vi "TCP-Get Status.vi"(0 "IP Address":string, 5 "Port":i32, 11 "error in (no error)":errorcluster) -> (4 "Recording":bool, 15 "error out":errorcluster)   [LabVIEW 2020]
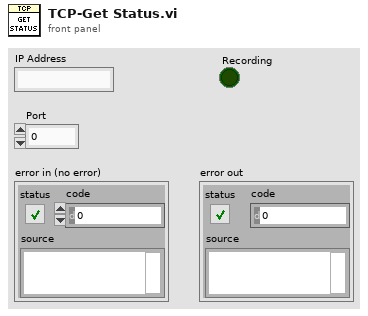
[diagram p1: front panel]
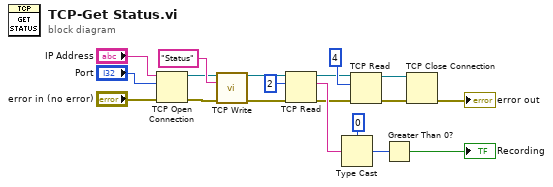
[diagram p0: block diagram]
diagram:
  n1 = TCP Open Connection(address="IP Address", remote port or service name="Port", error in (no error)="error in (no error)") -> (connection ID=w4:refnum<k5>, error out=w3:errorcluster)  [unwired: 2 in]
  n2 = call "TCP Write.vi"("connection ID"=w4, "data string"="Status", "error in (no error)"=w3) -> ("connection ID out"=w7:refnum<k5>, "error out"=w6:errorcluster)  [unwired: 10 in, 1 out]
  n3 = TCP Read(connection ID=w7, bytes to read=2, error in (no error)=w6) -> (connection ID out=w11:refnum<k5>, data out=w12:string, error out=w10:errorcluster)  [unwired: 2 in]
  n4 = Type Cast(type=i16 0, x=w12) -> (*(type *) &x=w17:i16)
  n5 = TCP Read(connection ID=w11, bytes to read=4, error in (no error)=w10) -> (connection ID out=w16:refnum<k5>, error out=w15:errorcluster)  [unwired: 2 in, 1 out]
  n6 = Greater Than 0?(x=w17) -> (x > 0?=→"Recording":bool)
  n7 = TCP Close Connection(connection ID=w16, error in (no error)=w15) -> (error out=→"error out":errorcluster)  [unwired: 1 in, 1 out]
